vi "Pendulum Stop.vi"(9 "timeout_sec":dbl, 10 "retry_mS":dbl, 11 "instance":i32) -> (3 "function return":i32)   [LabVIEW 2025, in "pendulumApp.lvlib"]
doc: "OOTB_API int Pendulum_Stop(int instance,double retry_mS);\n\nOOTB_API int Pendulum_Stop(int instance,double retry_mS, double timeout_sec);"
uses:
  pendulumApp.lvlib
  pendulumApp.dll
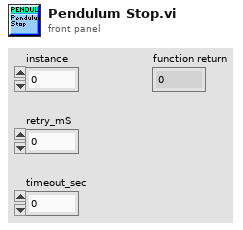
[diagram p1: front panel]
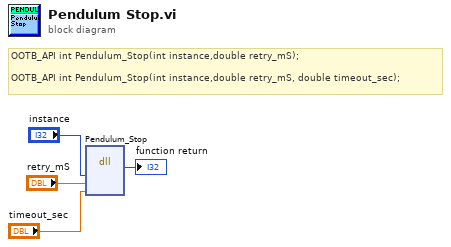
[diagram p0: block diagram]
diagram:
  # "OOTB_API\tint Pendulum_Stop(int instance,double retry_mS);\n\nOOTB_API\tint Pendulum_Stop(int instance,double retry_mS, double timeout_sec);"
  n1 = dll-call lib="C:/Users/noaht/School/Fall 2025/Controls Lab/Lab 4/FA25_pend_Lab3_4/SADI_Pendulum_lib/pendulumApp.*" fn="Pendulum_Stop"("instance"="instance", "retry_mS"="retry_mS", "timeout_sec"="timeout_sec") -> (→"function return":i32)  [unwired: 6 in, 2 out]
